vi "ATS_AsyncDMA_Device.vi"(0 "DeviceIn":i32, 1 "ATS_Async_Ctrl":T6, 5 "Async_Mode":T2, 7 "Async_Setting":T1, 9 "Channel":T7, 11 "ReadSamples":T4, 12 "Start Now / Wait":bool=TRUE, 13 "WaitTimeOut (ms)":u32=5000) -> (4 "Buffer":u16[](array[numeric]), 6 "Async_Status":T5, 10 "ReadSamples_Out":T4, 14 "cFlags_Out":u32 format="%x", 15 "Return Code":u32)   [LabVIEW 2010]
doc: "_____AlazarTech, Scope_____\n\nControl of the AsyncDMA configuration.\nMaster/Slave or Multi board configuration."
uses:
  ATS_ctl/ATS_DMA_Channel.ctl
  ATS_ctl/ATS_ReadSamples.ctl
  ATS_ctl/ATS_Async_Ctrl.ctl
  ATS_ctl/ATS_Async_Status.ctl
  ATS_ctl/ATS_AsyncDMA_cFlags_Opt.ctl
  ATS_ctl/ATS_Async_Mode.ctl
  ATS_ctl/ATS_Async_Setting.ctl
  ATS_ctl/ATS_Sys_Info.ctl
  ATS_ctl/ATS_Global_Ctrl.ctl
panel:
  out "CFlag_Option_Display":T3
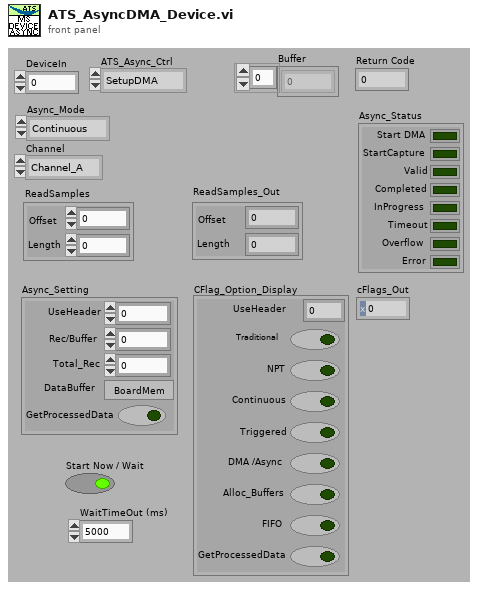
[diagram p1: front panel]
types:
  T1 = typedef "ATS_Async_Setting.ctl" = cluster{"UseHeader":u32, "Rec/Buffer":u32, "Total_Rec":u32, "DataBuffer":bool, "GetProcessedData":bool}
  T2 = typedef "ATS_Async_Mode.ctl" = enum16{"Continuous", "Triggered", "No-Pre-Trigger", "Traditional"}
  T3 = typedef "ATS_AsyncDMA_cFlags_Opt.ctl" = cluster{"UseHeader":u32, "Traditional":bool, "NPT":bool, "Continuous":bool, "Triggered":bool, "DMA /Async":bool, "Alloc_Buffers":bool, "FIFO":bool, "GetProcessedData":bool}
  T4 = typedef "ATS_ReadSamples.ctl" = cluster{"Offset":i32, "Length":u32}
  T5 = typedef "ATS_Async_Status.ctl" = cluster{"Start DMA":bool, "StartCapture":bool, "Valid":bool, "Completed":bool, "InProgress":bool, "Timeout":bool, "Overflow":bool, "Error":bool}
  T6 = typedef "ATS_Async_Ctrl.ctl" = enum16{"SetupDMA", "StartCapture", "Get", "Get_Stream", "Abort", "Stop"}
  T7 = typedef "ATS_DMA_Channel.ctl" = enum16{"Channel_A", "Channel_B", "A & B"}
  T8 = typedef "ATS_Sys_Info.ctl" = cluster{"MS_Mode":bool, "MBoard":i32, "#Board":i32}
  T9 = cluster{"UseHeader":u32, "HandleOut":u32, "ReadSamples_Out":T4, "BufferSize_Byte":u32, "First Call":bool, "TotalRecords":u32, "BufferSize_Sample":u32, "Buffer_Active":i32, "TimeOut (ms)":u32, "ActualRecord":u32, "Record/Buffer":u32, "Async_Status":T5, "Sys_Out":T8}
  T10 = typedef "ATS_Global_Ctrl.ctl" = enum16{"Init_Device", "Clear_ALL", "Set", "Get"}
  T11 = cluster{"UseHeader":u32, "HandleOut":u32, "ReadSamples_Out":T4, "BufferSize_Byte":u32, "First Call":bool, "TotalRecords":u32, "BufferSize_Sample":u32, "Buffer_Active":i32, "TimeOut (ms)":u32, "ActualRecord":u32, "Record/Buffer":u32, "Async_Status":T5, "Sys_Out":T8}[]
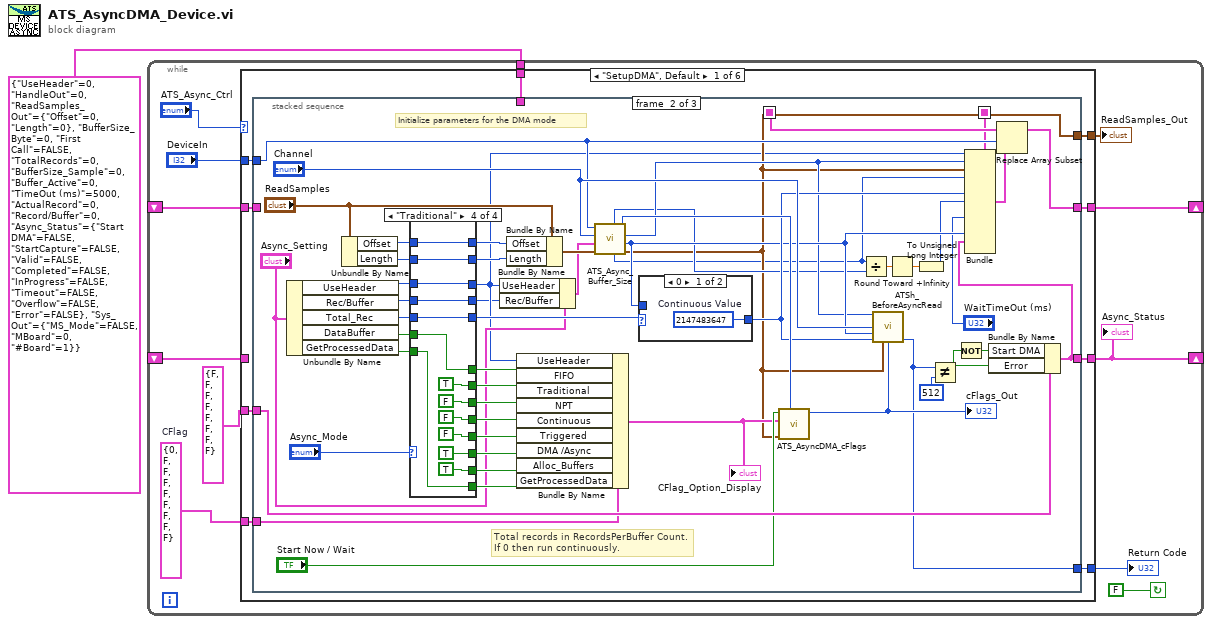
[diagram p0: block diagram]
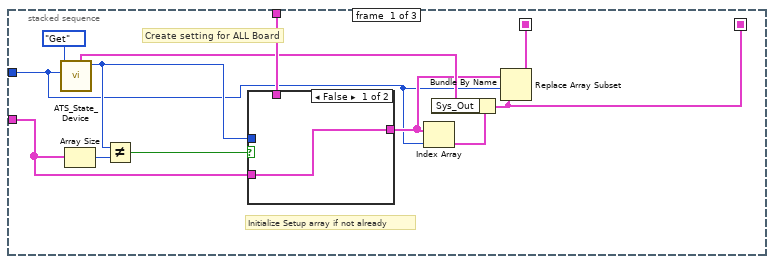
[diagram p2: hidden frame]
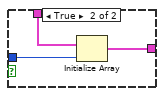
[diagram p3: hidden frame]
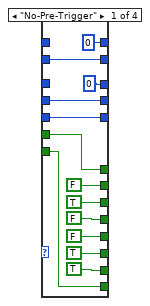
[diagram p4: hidden frame]
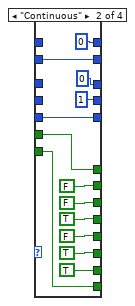
[diagram p5: hidden frame]
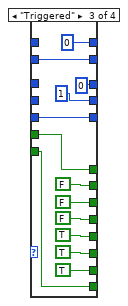
[diagram p6: hidden frame]
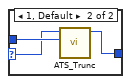
[diagram p7: hidden frame]
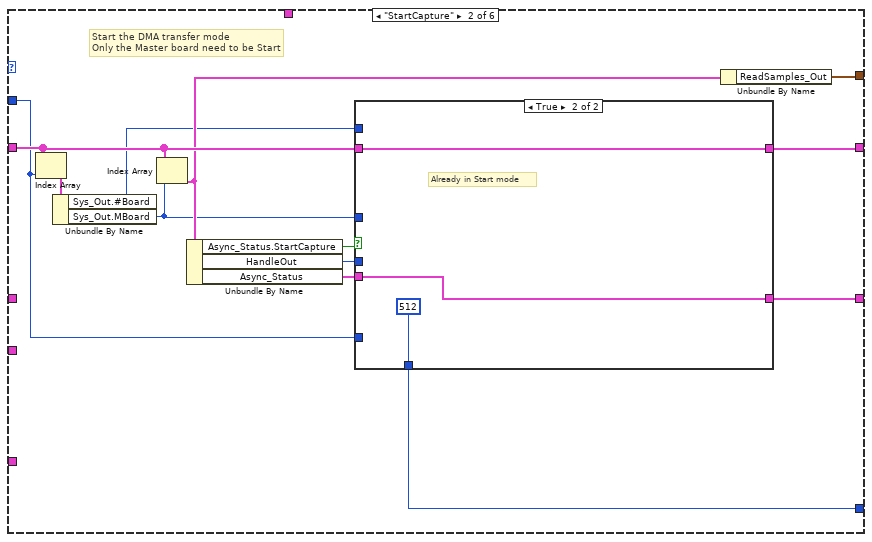
[diagram p9: hidden frame]
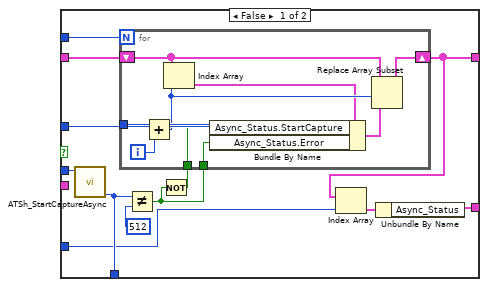
[diagram p10: hidden frame]
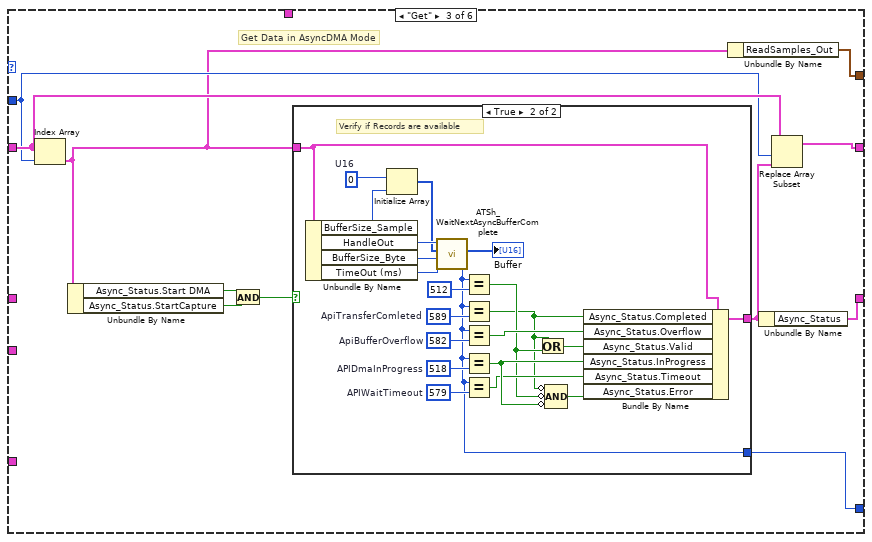
[diagram p11: hidden frame]
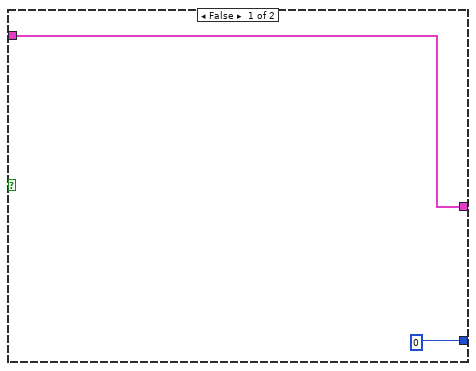
[diagram p12: hidden frame]
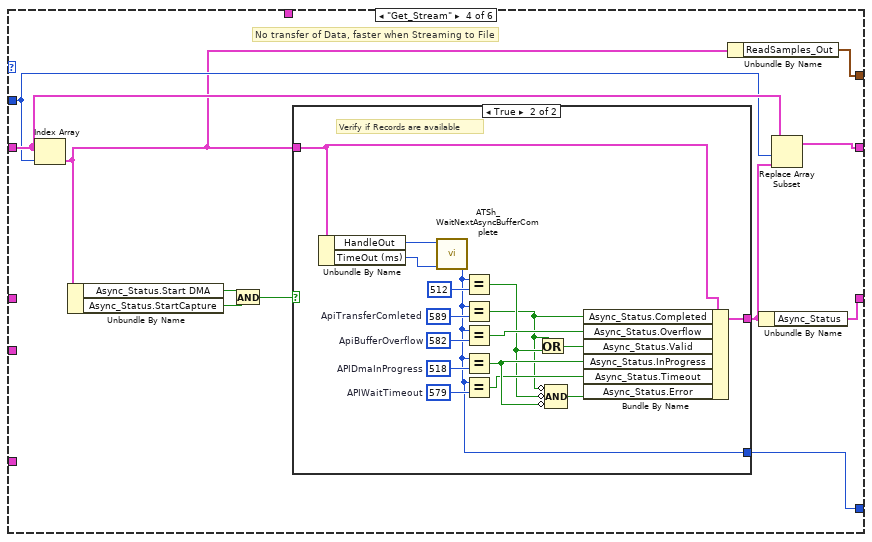
[diagram p13: hidden frame]
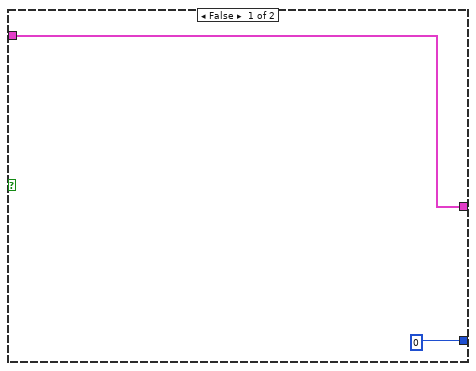
[diagram p14: hidden frame]
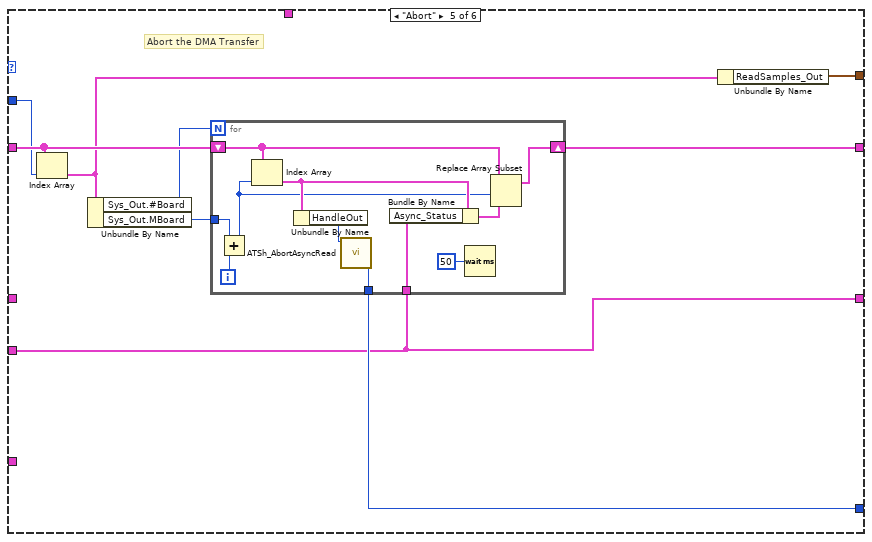
[diagram p15: hidden frame]
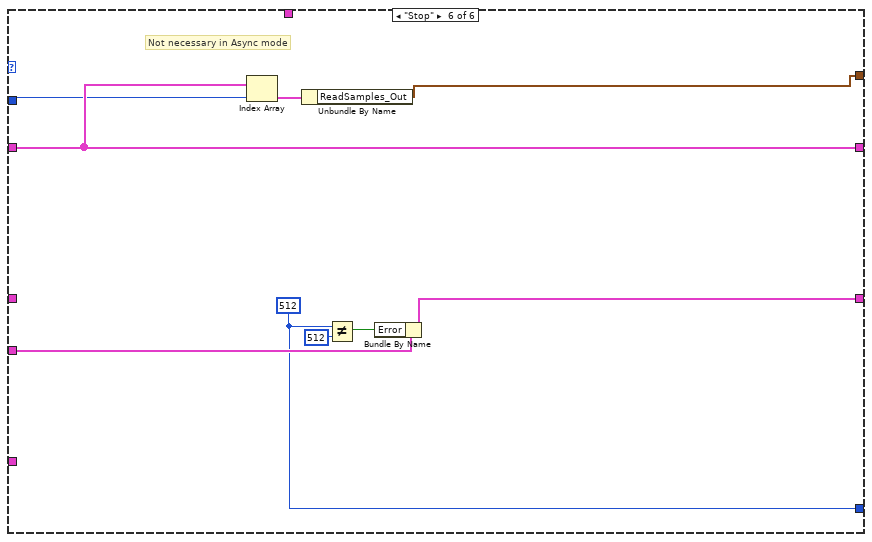
[diagram p16: hidden frame]
diagram:
  n1 = while {
    shift-right: [w8] -> _
    shift-left: _ -> [w10]
    shift-right: [w6] -> _
    shift-left: _ -> [w9]
    tunnel: T9 {"UseHeader"=0, "HandleOut"=0, "ReadSamples_Out"={"Offset"=0, "Length"=0}, "BufferSize_Byte"=0, "First Call"=FALSE, "TotalRecords"=0, "BufferSize_Sample"=0, "Buffer_Active"=0, "TimeOut (ms)"=5000, "ActualRecord"=0, "Record/Buffer"=0, "Async_Status"={"Start DMA"=FALSE, "StartCapture"=FALSE, "Valid"=FALSE, "Completed"=FALSE, "InProgress"=FALSE, "Timeout"=FALSE, "Overflow"=FALSE, "Error"=FALSE}, "Sys_Out"={"MS_Mode"=FALSE, "MBoard"=0, "#Board"=1}} -> [w7]
    stop <- FALSE continue-if-true
    w4 = T3 {"UseHeader"=0, "Traditional"=FALSE, "NPT"=FALSE, "Continuous"=FALSE, "Triggered"=FALSE, "DMA /Async"=FALSE, "Alloc_Buffers"=FALSE, "FIFO"=FALSE, "GetProcessedData"=FALSE}  # CFlag
    n2 = case shown="\"SetupDMA\", Default" "ATS_Async_Ctrl" {
      tunnel: [w20 w152 w187 w222 w254 w272] -> w8
      tunnel: [w18 w159 w194 w229 w257 w273] -> w11
      tunnel: w10 -> [w15 w154 w191 w226 w255 w272]
      tunnel: [w21 w157 w189 w224 w256 w277] -> w6
      tunnel: w9 -> [_ _ _ _ _ _]
      tunnel: T5 {"Start DMA"=FALSE, "StartCapture"=FALSE, "Valid"=FALSE, "Completed"=FALSE, "InProgress"=FALSE, "Timeout"=FALSE, "Overflow"=FALSE, "Error"=FALSE} ("Async_Status") -> [w22 _ _ _ w256 w274]
      tunnel: w7 -> [w19 _ _ _ _ _]
      tunnel: w4 -> [w17 _ _ _ _ _]
      tunnel: "DeviceIn" -> [w16 w147 w190 w225 w249 w271]
      tunnel: [w14 w156 w185 w220 w253 w269] -> w2
      frame "SetupDMA", Default {
        n3 = stacked-sequence {
          seq-local: [w25 _ _] -> [_ w64 _]
          seq-local: [w23 _ _] -> [_ w39 _]
          tunnel: w22 -> [_ w90 _]
          tunnel: [_ w62 _] -> w21
          tunnel: [_ w57 _] -> w20
          tunnel: w19 -> [w32 _ _]
          tunnel: [_ w81 _] -> w18
          tunnel: w17 -> [_ w68 _]
          tunnel: w16 -> [w24 w56 _]
          tunnel: w15 -> [w30 _ _]
          tunnel: [_ w54 _] -> w14
          frame #0 {
            # "Create setting for ALL Board"
            # "Initialize Setup array if not already"
            n4 = call "ATS_State_Device.vi"("DeviceIn"=w24, "ATS_GBL_Ctrl"=ATS_Global_Ctrl."Get") -> ("#Device"=w27:i32, "Sys_Out"=w28:T8)  [unwired: 4 in, 4 out]
            n5 = Array Size(array=w30) -> (size(s)=w33:i32)
            n6 = Not Equal?(x=w27, y=w33) -> (x != y?=w31:bool)
            n7 = case shown="False" w31 {
              tunnel: w27 -> [_ w36]
              tunnel: w32 -> [_ w38]
              tunnel: [w35 w37] -> w26
              tunnel: w30 -> [w35 _]
              frame False {
              }
              frame True {
                n8 = Initialize Array(w38, w36) -> (w37:T11)
              }
            }
            n9 = Index Array(array=w26, index=w24) -> (element=w29:T9)
            n10 = Bundle By Name(cluster=w29, "Sys_Out"=w28) -> (w23:T9)
            n11 = Replace Array Subset(array=w26, new element=w23, index=w24) -> (w25:T11)
          }
          frame #1 {
            # "Total records in RecordsPerBuffer Count.\nIf 0 then run continuously."
            # "Initialize parameters for the DMA mode"
            n12 = Unbundle By Name("Async_Setting") -> ("UseHeader"=w48:u32, "Rec/Buffer"=w49:u32, "Total_Rec"=w50:u32, "DataBuffer"=w51:bool, "GetProcessedData"=w52:bool)
            n13 = Unbundle By Name("ReadSamples") -> ("Offset"=w45:i32, "Length"=w46:u32)
            n14 = case shown="\"Traditional\"" "Async_Mode" {
              tunnel: [u32 0 u32 0 u32 0 w132] -> w42
              tunnel: [0 ("Offset") 0 ("Offset") 0 ("Offset") w130] -> w78
              tunnel: [w95 w107 w120 w131] -> w76
              tunnel: [w91 u32 1 ("Rec/Buffer") u32 1 ("Rec/Buffer") w133] -> w40
              tunnel: [w92 w106 w119 w134] -> w77
              tunnel: [FALSE ("DMA /Async") TRUE ("DMA /Async") FALSE ("DMA /Async") FALSE ("DMA /Async")] -> w75
              tunnel: [TRUE ("Trig_Stream") FALSE ("Trig_Stream") FALSE ("Trig_Stream") FALSE ("Trig_Stream")] -> w74
              tunnel: [FALSE ("Trig_Stream") FALSE ("Trig_Stream") FALSE ("Trig_Stream") TRUE ("Trig_Stream")] -> w73
              tunnel: [TRUE ("DMA /Async") TRUE ("DMA /Async") TRUE ("DMA /Async") TRUE ("DMA /Async")] -> w72
              tunnel: [FALSE ("DMA /Async") FALSE ("DMA /Async") TRUE ("DMA /Async") FALSE ("DMA /Async")] -> w71
              tunnel: [TRUE ("DMA /Async") TRUE ("DMA /Async") TRUE ("DMA /Async") TRUE ("DMA /Async")] -> w69
              tunnel: [w93 w105 w118 w135] -> w65
              tunnel: [w94 w104 w117 w136] -> w53
              tunnel: w52 -> [w94 w104 w117 w136]
              tunnel: w51 -> [w93 w105 w118 w135]
              tunnel: w50 -> [w92 w106 w119 w134]
              tunnel: w49 -> [w91 _ _ w133]
              tunnel: w48 -> [_ _ _ w132]
              tunnel: w46 -> [w95 w107 w120 w131]
              tunnel: w45 -> [_ _ _ w130]
              frame "No-Pre-Trigger" {
              }
              frame "Continuous" {
              }
              frame "Triggered" {
              }
              frame "Traditional" {
              }
            }
            n15 = Bundle By Name(cluster="Async_Setting", "UseHeader"=w42, "Rec/Buffer"=w40) -> (w41:T1)
            n16 = Bundle By Name(cluster="ReadSamples", "Offset"=w78, "Length"=w76) -> (w55:T4)
            n17 = Bundle By Name(cluster=w68, "UseHeader"=w42, "FIFO"=w65, "Traditional"=w73, "NPT"=w74, "Continuous"=w75, "Triggered"=w71, "DMA /Async"=w72, "Alloc_Buffers"=w69, "GetProcessedData"=w53) -> (w79:T3)
            "CFlag_Option_Display" <- w79
            n18 = call "ATS_Async_Buffer_Size.vi"("ReadSamples"=w55, "Async_Setting"=w41, "Channel"="Channel", "DeviceIn"=w56) -> ("ReadSamples_Out"=w54:T4, "RecordsPerBuffer_Out"=w70:u32, "Handle"=w67:u32, "DeviceOut"=w85:i32, "BufferSize"=w44:u32, "#Bytes/Sample"=w61:u32)  [unwired: 2 in]
            n19 = case shown="0" w77 {
              selector: w77 -> [_ w144]
              tunnel: w70 -> [_ w146]
              tunnel: [w143 w145] -> w82
              frame 0 {
                w143 = u32 2147483647  # Continuous Value
              }
              frame 1, Default {
                n20 = call "ATS_Trunc.vi"("TruncValue"=w146, "Value"=w144) -> ("NewValue"=w145:u32)  [unwired: 5 in]
              }
            }
            n21 = call "ATS_AsyncDMA_cFlags.vi"("DeviceIn"=w85, "ReadSamples"=w54, "cFlags_Options"=w79, "Start Now / Wait"="Start Now / Wait") -> ("cFlags_Out"=w83:u32)  [unwired: 6 in, 1 out]
            "cFlags_Out" <- w83
            n22 = Divide(x=w44, y=w61) -> (x/y=w60:dbl)
            n23 = call "ATSh_BeforeAsyncRead.vi"("Handle"=w67, "Channel"="Channel", "RecordsPerBuffer"=w70, "RecordsCount"=w82, "ReadSamples"=w54, "cFlags"=w83) -> ("Return Code"=w81:u32)  [unwired: 8 in, 1 out]
            n24 = Round Toward +Infinity(x=w60) -> (ceil(x): smallest int >= x=w59:dbl)
            n25 = To Unsigned Long Integer(number=w59) -> (unsigned 32bit integer=w58:u32)
            n26 = Not Equal?(x=w81, y=u32 512 ("x")) -> (x != y?=w88:bool)
            n27 = Not(x=w88) -> (.not. x?=w87:bool)
            n28 = Bundle By Name(cluster=w90, "Start DMA"=w87, "Error"=w88) -> (w62:T5)
            n29 = Bundle(cluster=w39, "UseHeader"=w42, "HandleOut"=w67, "ReadSamples_Out"=w54, "BufferSize_Byte"=w44, "TotalRecords"=w82, "BufferSize_Sample"=w58, "TimeOut (ms)"="WaitTimeOut (ms)", "Record/Buffer"=w70, "Async_Status"=w62) -> (w63:T9)  [unwired: 4 in]
            n30 = Replace Array Subset(array=w64, new element=w63, index=w56) -> (w57:T11)
          }
          frame #2 {
          }
        }
      }
      frame "StartCapture" {
        # "Start the DMA transfer mode\nOnly the Master board need to be Start"
        n31 = Index Array(array=w154, index=w147) -> (element=w155:T9)
        n32 = Unbundle By Name(w155) -> ("Sys_Out.#Board"=w150:i32, "Sys_Out.MBoard"=w151:i32)
        n33 = Index Array(array=w154, index=w151) -> (element=w153:T9)
        n34 = Unbundle By Name(w153) -> ("Async_Status.StartCapture"=w149:bool, "HandleOut"=w158:u32, "Async_Status"=w148:T5)
        n35 = case shown="True" w149 {
          tunnel: [w171 u32 512 ("Return Code")] -> w159
          tunnel: w158 -> [w169 _]
          tunnel: [w168 w181] -> w157
          tunnel: w154 -> [w167 w182]
          tunnel: [w161 w182] -> w152
          tunnel: w151 -> [w166 _]
          tunnel: w150 -> [w165 _]
          tunnel: w148 -> [_ w181]
          tunnel: w147 -> [w160 _]
          frame False {
            n36 = call "ATSh_StartCaptureAsync.vi"("Handle"=w169) -> ("Return Code"=w171:u32)  [unwired: 10 in]
            n37 = Not Equal?(x=w171, y=u32 512) -> (x != y?=w164:bool)
            n38 = Not(x=w164) -> (.not. x?=w163:bool)
            n39 = for {
              N: w165 -> [_]
              shift-right: [w180] -> w161
              shift-left: w167 -> [w177]
              tunnel: w166 -> [w179]
              tunnel: w164 -> [w173]
              tunnel: w163 -> [w172]
              i -> [w178]
              n40 = Add(x=w179, y=w178) -> (x+y=w176:i32)
              n41 = Index Array(array=w177, index=w176) -> (element=w175:T9)
              n42 = Bundle By Name(cluster=w175, "Async_Status.StartCapture"=w172, "Async_Status.Error"=w173) -> (w174:T9)
              n43 = Replace Array Subset(array=w177, new element=w174, index=w176) -> (w180:T11)
            }
            n44 = Index Array(array=w161, index=w160) -> (element=w162:T9)
            n45 = Unbundle By Name(w162) -> ("Async_Status"=w168:T5)
          }
          frame True {
            # "Already in Start mode"
          }
        }
        n46 = Unbundle By Name(w153) -> ("ReadSamples_Out"=w156:T4)
      }
      frame "Get" {
        # "Get Data in AsyncDMA Mode"
        n47 = Index Array(array=w191, index=w190) -> (element=w186:T9)
        n48 = Unbundle By Name(w186) -> ("Async_Status.Start DMA"=w193:bool, "Async_Status.StartCapture"=w192:bool)
        n49 = And(x=w193, y=w192) -> (x .and. y?=w184:bool)
        n50 = case shown="True" w184 {
          tunnel: [w195 w218] -> w188
          tunnel: [u32 0 ("Return Code") w204] -> w194
          tunnel: w186 -> [w195 w205]
          frame False {
          }
          frame True {
            w199 = u16 0  # U16
            w209 = u32 589  # ApiTransferComleted
            w212 = u32 582  # ApiBufferOverflow
            w215 = u32 579  # APIWaitTimeout
            w216 = u32 518  # APIDmaInProgress
            # "Verify if Records are available"
            n51 = Unbundle By Name(w205) -> ("BufferSize_Sample"=w198:u32, "HandleOut"=w201:u32, "BufferSize_Byte"=w203:u32, "TimeOut (ms)"=w202:u32)
            n52 = Initialize Array(w199, w198) -> (w197:u16[])
            n53 = call "ATSh_WaitNextAsyncBufferComplete.vi"("uTimeout_ms"=w202, "uBytesPerBuffer"=w203, "pBuffer_In"=w197, "Handle"=w201) -> ("Return Code"=w204:u32, "pBuffer_Out"=→"Buffer":u16[])  [unwired: 5 in, 1 out]
            n54 = Equal?(x=w204, y=u32 512 ("x")) -> (x = y?=w207:bool)
            n55 = Equal?(x=w204, y=w209) -> (x = y?=w206:bool)
            n56 = Equal?(x=w204, y=w212) -> (x = y?=w211:bool)
            n57 = Equal?(x=w204, y=w216) -> (x = y?=w214:bool)
            n58 = Equal?(x=w204, y=w215) -> (x = y?=w213:bool)
            n59 = Or(x=w206, y=w207) -> (x .or. y?=w208:bool)
            n60 = Compound Arithmetic op=AND(invert w206, invert w207, invert w214) -> (w210:bool)
            n61 = Bundle By Name(cluster=w205, "Async_Status.Completed"=w206, "Async_Status.Overflow"=w211, "Async_Status.Valid"=w208, "Async_Status.InProgress"=w214, "Async_Status.Timeout"=w213, "Async_Status.Error"=w210) -> (w218:T9)
          }
        }
        n62 = Unbundle By Name(w186) -> ("ReadSamples_Out"=w185:T4)
        n63 = Unbundle By Name(w188) -> ("Async_Status"=w189:T5)
        n64 = Replace Array Subset(array=w191, new element=w188, index=w190) -> (w187:T11)
      }
      frame "Get_Stream" {
        # "No transfer of Data, faster when Streaming to File"
        n65 = Index Array(array=w226, index=w225) -> (element=w221:T9)
        n66 = Unbundle By Name(w221) -> ("Async_Status.Start DMA"=w228:bool, "Async_Status.StartCapture"=w227:bool)
        n67 = And(x=w228, y=w227) -> (x .and. y?=w219:bool)
        n68 = case shown="True" w219 {
          tunnel: [w230 w248] -> w223
          tunnel: [u32 0 ("Return Code") w234] -> w229
          tunnel: w221 -> [w230 w235]
          frame False {
          }
          frame True {
            w239 = u32 589  # ApiTransferComleted
            w242 = u32 582  # ApiBufferOverflow
            w245 = u32 579  # APIWaitTimeout
            w246 = u32 518  # APIDmaInProgress
            # "Verify if Records are available"
            n69 = Unbundle By Name(w235) -> ("HandleOut"=w232:u32, "TimeOut (ms)"=w233:u32)
            n70 = call "ATSh_WaitNextAsyncBufferComplete.vi"("uTimeout_ms"=w233, "Handle"=w232) -> ("Return Code"=w234:u32)  [unwired: 7 in, 2 out]
            n71 = Equal?(x=w234, y=u32 512 ("x")) -> (x = y?=w237:bool)
            n72 = Equal?(x=w234, y=w239) -> (x = y?=w236:bool)
            n73 = Equal?(x=w234, y=w242) -> (x = y?=w241:bool)
            n74 = Equal?(x=w234, y=w246) -> (x = y?=w244:bool)
            n75 = Equal?(x=w234, y=w245) -> (x = y?=w243:bool)
            n76 = Or(x=w236, y=w237) -> (x .or. y?=w238:bool)
            n77 = Compound Arithmetic op=AND(invert w236, invert w237, invert w244) -> (w240:bool)
            n78 = Bundle By Name(cluster=w235, "Async_Status.Completed"=w236, "Async_Status.Overflow"=w241, "Async_Status.Valid"=w238, "Async_Status.InProgress"=w244, "Async_Status.Timeout"=w243, "Async_Status.Error"=w240) -> (w248:T9)
          }
        }
        n79 = Unbundle By Name(w221) -> ("ReadSamples_Out"=w220:T4)
        n80 = Unbundle By Name(w223) -> ("Async_Status"=w224:T5)
        n81 = Replace Array Subset(array=w226, new element=w223, index=w225) -> (w222:T11)
      }
      frame "Abort" {
        # "Abort the DMA Transfer"
        n82 = Index Array(array=w255, index=w249) -> (element=w252:T9)
        n83 = Unbundle By Name(w252) -> ("Sys_Out.#Board"=w251:i32, "Sys_Out.MBoard"=w250:i32)
        n84 = for {
          N: w251 -> [_]
          tunnel: [w267] -> w257
          tunnel: w256 -> [w266]
          shift-right: [w264] -> w254
          shift-left: w255 -> [w263]
          tunnel: w250 -> [w259]
          i -> [w260]
          n85 = Add(x=w259, y=w260) -> (x+y=w258:i32)
          n86 = Index Array(array=w263, index=w258) -> (element=w262:T9)
          n87 = Unbundle By Name(w262) -> ("HandleOut"=w268:u32)
          n88 = call "ATSh_AbortAsyncRead.vi"("Handle"=w268) -> ("Return Code"=w267:u32)  [unwired: 10 in]
          n89 = Bundle By Name(cluster=w262, "Async_Status"=w266) -> (w265:T9)
          n90 = Wait (ms)(milliseconds to wait=u32 50) -> ()  [unwired: 1 out]
          n91 = Replace Array Subset(array=w263, new element=w265, index=w258) -> (w264:T11)
        }
        n92 = Unbundle By Name(w252) -> ("ReadSamples_Out"=w253:T4)
      }
      frame "Stop" {
        w273 = u32 512 ("Return Code")
        # "Not necessary in Async mode"
        n93 = Index Array(array=w272, index=w271) -> (element=w270:T9)
        n94 = Unbundle By Name(w270) -> ("ReadSamples_Out"=w269:T4)
        n95 = Not Equal?(x=w273, y=u32 512) -> (x != y?=w276:bool)
        n96 = Bundle By Name(cluster=w274, "Error"=w276) -> (w277:T5)
      }
    }
    "Return Code" <- w11
    "Async_Status" <- w6
    "ReadSamples_Out" <- w2
  }
